vi "count types.vi"() -> (3 "type count":i32)   [LabVIEW 2013, in "data bus tag description.lvclass"]
doc: "Indicates the number of types supported by the framework."
uses:
  data bus tag description.lvclass
  Data Type.ctl
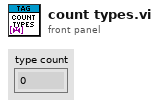
[diagram p1: front panel]
types:
  T1 = typedef "data bus tag description.lvclass/Data Type.ctl" = enum16{"Double", "I64", "Boolean", "Array of Double", "Array of I64", "Variant"}
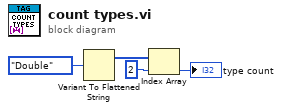
[diagram p0: block diagram]
diagram:
  n1 = Variant To Flattened String(Variant=Data_Type."Double" ("Data Type")) -> (1:w4:i16[])  [unwired: 1 out]
  n2 = Index Array(array=w4, index=2) -> (element=→"type count":i16)
